vi "PAN_MacroMgr.vi"(10 "macrodir":path) -> ()   [LabVIEW 2016]
panel:
  in  "Cluster":T1
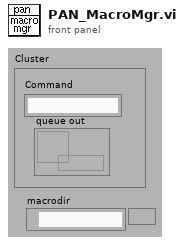
[diagram p1: front panel]
types:
  T1 = cluster{"Command ":string, "queue out":refnum<queue>}
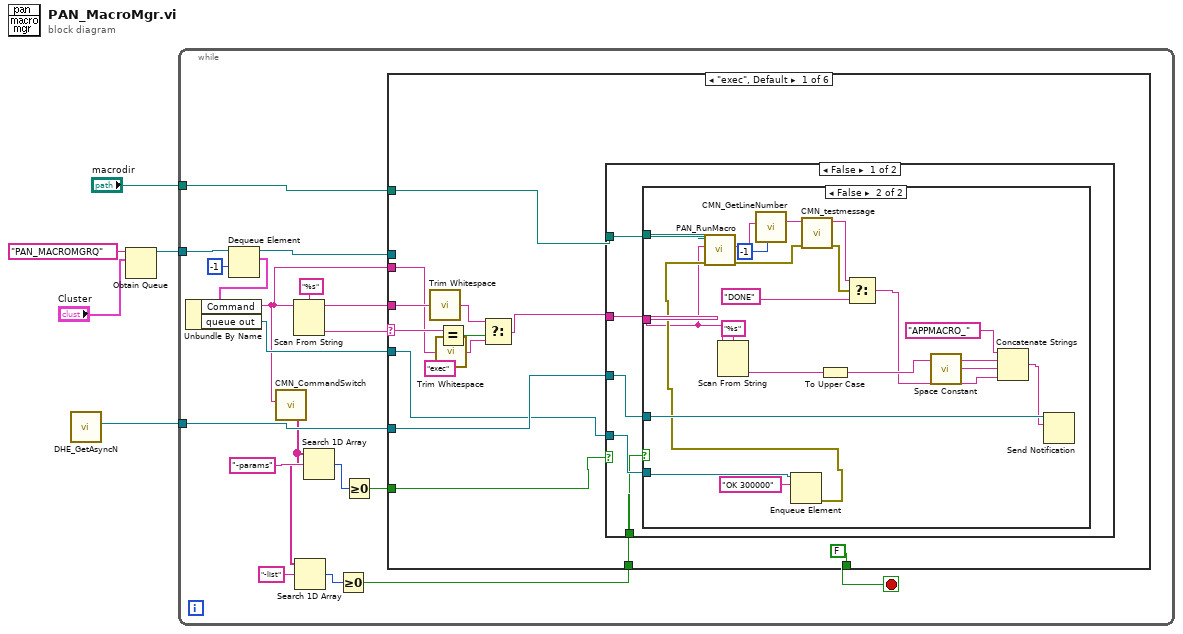
[diagram p0: block diagram]
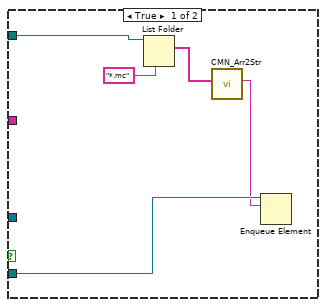
[diagram p2: hidden frame]
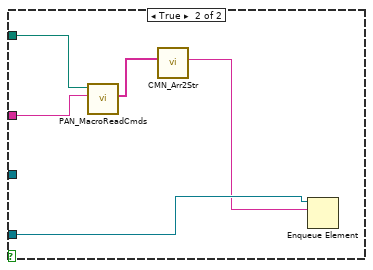
[diagram p3: hidden frame]
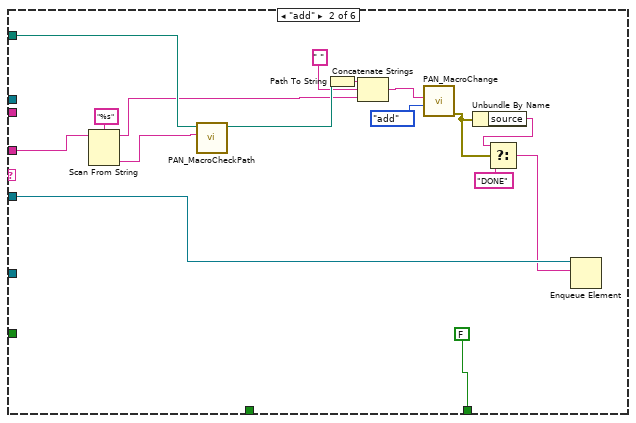
[diagram p4: hidden frame]
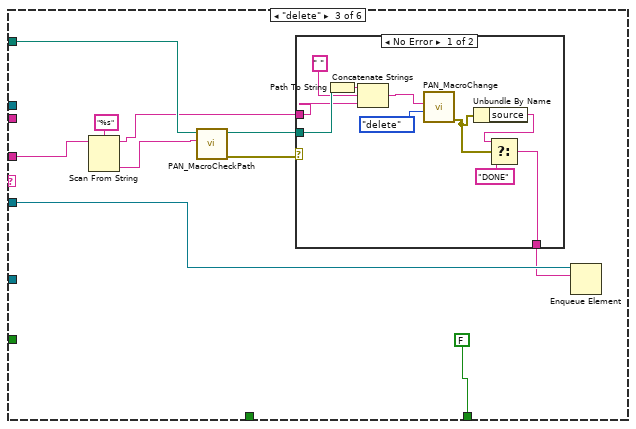
[diagram p5: hidden frame]
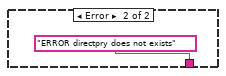
[diagram p6: hidden frame]
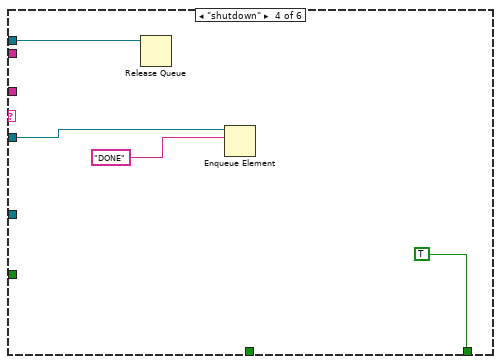
[diagram p7: hidden frame]
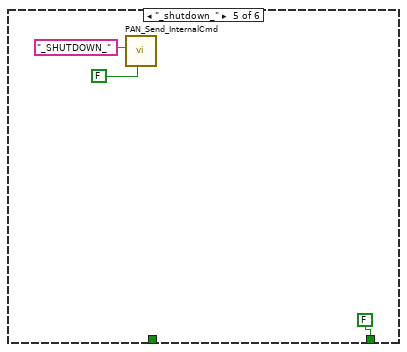
[diagram p8: hidden frame]
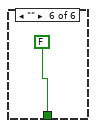
[diagram p9: hidden frame]
diagram:
  n1 = call "DHE_GetAsyncN.vi"() -> ("asyncN"=w3:refnum<notifier>)  [unwired: 11 out]
  n2 = Obtain Queue(name (unnamed)="PAN_MACROMGRQ", element data type="Cluster") -> (queue out=w5:refnum<queue>)  [unwired: 3 in, 2 out]
  n3 = while {
    tunnel: w5 -> [w24]
    tunnel: w3 -> [w17]
    tunnel: "macrodir" -> [w14]
    stop <- w21 stop-if-true
    n4 = Dequeue Element(queue=w24, timeout in ms (-1)=-1) -> (queue out=w18:refnum<queue>, element=w16:T1)  [unwired: 1 in, 2 out]
    n5 = Unbundle By Name(w16) -> ("Command"=w6:string, "queue out"=w15:refnum<queue>)
    n6 = call "CMN_CommandSwitch.vi"("command in"=w6) -> ("swhitches"=w10:string[])  [unwired: 1 in, 9 out]
    n7 = Scan From String(format string="%s", input string=w6) -> (remaining string=w19:string, output 1=w22:string)  [unwired: 2 in, 3 out]
    n8 = Search 1D Array(1D array=w10, element="-list") -> (index of element=w8:i32)  [unwired: 1 out]
    n9 = Search 1D Array(1D array=w10, element="-params") -> (index of element=w12:i32)  [unwired: 1 out]
    n10 = Greater Or Equal To 0?(x=w8) -> (x >= 0?=w7:bool)
    n11 = Greater Or Equal To 0?(x=w12) -> (x >= 0?=w11:bool)
    n12 = case shown="\"exec\", Default" w22 {
      selector: w22 -> [w35 _ _ _ _ _]
      tunnel: [FALSE FALSE FALSE TRUE FALSE FALSE] -> w21
      tunnel: w19 -> [w34 w82 w95 _ _ _]
      tunnel: w18 -> [_ _ _ w113 _ _]
      tunnel: w17 -> [w32 _ _ _ _ _]
      tunnel: w15 -> [w31 w88 w98 w112 _ _]
      tunnel: w14 -> [w28 w84 w93 _ _ _]
      tunnel: w11 -> [w30 _ _ _ _ _]
      tunnel: w7 -> [w29 _ _ _ _ _]
      tunnel: w6 -> [w26 _ _ _ _ _]
      frame "exec", Default {
        n13 = call <vilib>:"Trim Whitespace.vi"("string"=w34) -> ("trimmed string"=w33:string)  [unwired: 1 in]
        n14 = call <vilib>:"Trim Whitespace.vi"("string"=w26) -> ("trimmed string"=w25:string)  [unwired: 1 in]
        n15 = Equal?(x=w35, y="exec") -> (x = y?=w37:bool)
        n16 = Select(t=w33, s=w37, f=w25) -> (s? t:f=w27:string)
        n17 = case shown="False" w30 {
          tunnel: w32 -> [w43 _]
          tunnel: w31 -> [w42 w73]
          tunnel: w29 -> [w41 _]
          tunnel: w28 -> [w40 w70]
          tunnel: w27 -> [w39 w71]
          frame False {
            n18 = case shown="False" w41 {
              tunnel: w43 -> [_ w68]
              tunnel: w42 -> [w46 w66]
              tunnel: w40 -> [w48 w56]
              tunnel: w39 -> [_ w55]
              frame True {
                n19 = List Folder(path=w48, pattern="*.mc") -> (filenames=w45:string[])  [unwired: 1 in, 4 out]
                n20 = call "CMN_Arr2Str.vi"("Array in"=w45) -> ("string out"=w44:string)  [unwired: 10 out]
                n21 = Enqueue Element(queue=w46, element=w44) -> ()  [unwired: 1 in, 4 out]
              }
              frame False {
                n22 = Scan From String(format string="%s", input string=w55) -> (output 1=w62:string)  [unwired: 2 in, 4 out]
                n23 = Enqueue Element(queue=w66, element="OK 300000") -> (error out=w59:errorcluster)  [unwired: 1 in, 3 out]
                n24 = call "PAN_RunMacro.vi"("error in (no error)"=w59, "commands"=w55, "macrodir"=w56) -> ("error out"=w51:errorcluster, "response"=w54:string)  [unwired: 7 out]
                n25 = call "CMN_GetLineNumber.vi"("line no"=-1, "multi-line string"=w54) -> ("line"=w52:string)  [unwired: 9 out]
                n26 = call "CMN_testmessage.vi"("error in (no error)"=w51, "message  in"=w52) -> ("error out"=w50:errorcluster, "message out"=w49:string)  [unwired: 8 out]
                n27 = To Upper Case(1:w62) -> (0:w61:string)
                n28 = Select(t=w49, s=w50, f="DONE") -> (s? t:f=w58:string)
                n29 = call <vilib>:"Space Constant.vi"() -> ("String"=w60:string)
                n30 = Concatenate Strings("APPMACRO_" ("string"), w61, w60, w58) -> (w67:string)
                n31 = Send Notification(notification=w67, notifier=w68) -> ()  [unwired: 1 in, 2 out]
              }
            }
          }
          frame True {
            n32 = call "PAN_MacroReadCmds.vi"("CommandStr"=w71, "macrodir"=w70) -> ("commands"=w69:string[])  [unwired: 9 out]
            n33 = call "CMN_Arr2Str.vi"("Array in"=w69) -> ("string out"=w72:string)  [unwired: 10 out]
            n34 = Enqueue Element(queue=w73, element=w72) -> ()  [unwired: 1 in, 4 out]
          }
        }
      }
      frame "add" {
        n35 = Scan From String(format string="%s", input string=w82) -> (remaining string=w81:string, output 1=w85:string)  [unwired: 2 in, 3 out]
        n36 = call "PAN_MacroCheckPath.vi"("CommandStr"=w85, "macrodir"=w84) -> ("output path"=w83:path)  [unwired: 9 out]
        n37 = Path To String(path=w83) -> (string=w79:string)
        n38 = Concatenate Strings(w79, " " ("string"), w81) -> (w77:string)
        n39 = call "PAN_MacroChange.vi"("action"=enum16{"add", "delete"}."add", "argument"=w77) -> ("error out"=w76:errorcluster)  [unwired: 1 in, 8 out]
        n40 = Unbundle By Name(w76) -> ("source"=w75:string)
        n41 = Select(t=w75, s=w76, f="DONE") -> (s? t:f=w87:string)
        n42 = Enqueue Element(queue=w88, element=w87) -> ()  [unwired: 1 in, 4 out]
      }
      frame "delete" {
        n43 = Scan From String(format string="%s", input string=w95) -> (remaining string=w90:string, output 1=w94:string)  [unwired: 2 in, 3 out]
        n44 = call "PAN_MacroCheckPath.vi"("CommandStr"=w94, "macrodir"=w93) -> ("error out"=w92:errorcluster, "output path"=w91:path)  [unwired: 8 out]
        n45 = case shown="No Error" w92 {
          tunnel: [w102 "ERROR directpry does not exists" ("source")] -> w97
          tunnel: w91 -> [w108 _]
          tunnel: w90 -> [w100 _]
          frame No Error {
            n46 = Path To String(path=w108) -> (string=w107:string)
            n47 = Concatenate Strings(w107, " " ("string"), w100) -> (w105:string)
            n48 = call "PAN_MacroChange.vi"("action"=enum16{"add", "delete"}."delete", "argument"=w105) -> ("error out"=w101:errorcluster)  [unwired: 1 in, 8 out]
            n49 = Unbundle By Name(w101) -> ("source"=w104:string)
            n50 = Select(t=w104, s=w101, f="DONE") -> (s? t:f=w102:string)
          }
          frame Error {
          }
        }
        n51 = Enqueue Element(queue=w98, element=w97) -> ()  [unwired: 1 in, 4 out]
      }
      frame "shutdown" {
        n52 = Release Queue(queue=w113) -> ()  [unwired: 1 in, 4 out]
        n53 = Enqueue Element(queue=w112, element="DONE" ("name (unnamed)")) -> ()  [unwired: 1 in, 4 out]
      }
      frame "_shutdown_" {
        n54 = call "PAN_Send_InternalCmd.vi"("wait response"=FALSE, "command"="_SHUTDOWN_") -> ()  [unwired: 3 in, 7 out]
      }
      frame "" {
      }
    }
  }
